vi "NI cDAQ-9188 Producer.vi"(7 "Control Notifier":refnum<notifier>, 8 "error in":errorcluster, 9 "Counter Task":refnum<k21>, 10 "AI Voltage Task":refnum<k21>, 11 "DAQ Notifier":refnum<notifier>) -> (0 "error out":errorcluster, 1 "Counter Task out":refnum<k21>, 2 "AI Voltage Task out":refnum<k21>, 3 "DAQ Notifier out":refnum<notifier>)   [LabVIEW 2013, in "Breakdown Acoustics Controls.lvlib"]
uses:
  Breakdown Acoustics Controls.lvlib
  <vilib>/DAQmx/read.llb/DAQmx Read (Analog 1D Wfm NChan NSamp).vi
  <resource>/objmgr/daqmx.rc
panel:
  in  "Samples per Channel":u32=5120
  in  "Sampling Rate (Hz)":u32=100000
  in  "Stop":bool
  out "ms since last read":u32
  out "Waveform Graph":waveform(dbl)[](graph)
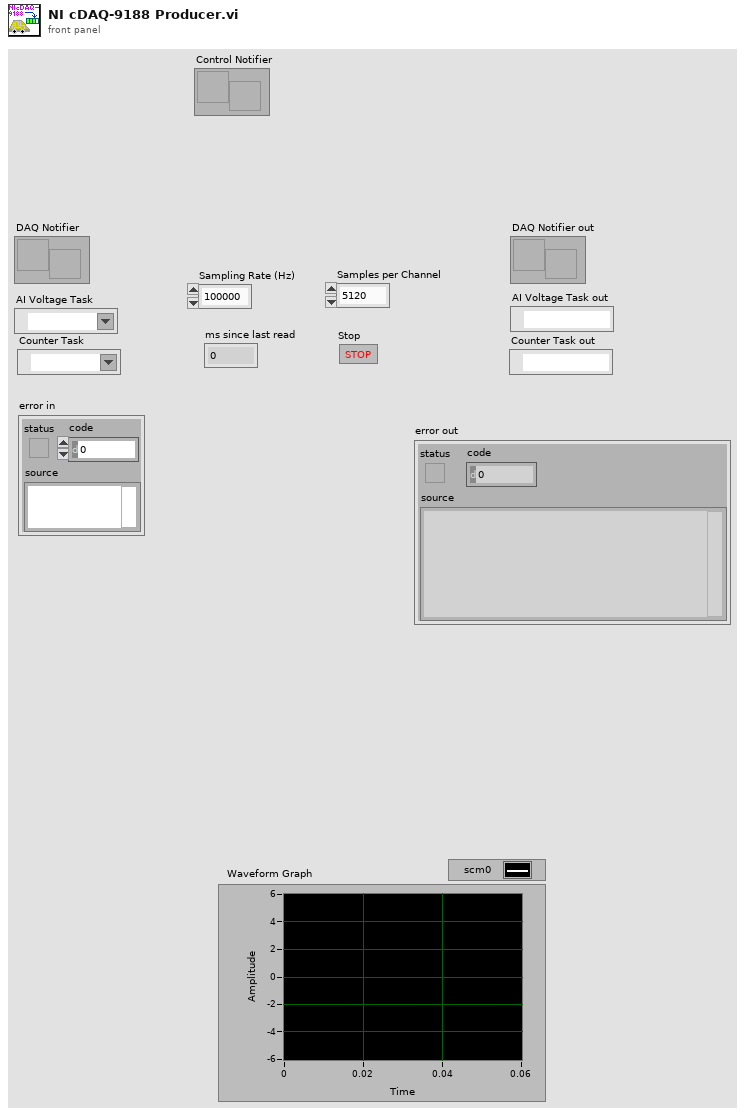
[diagram p1: front panel]
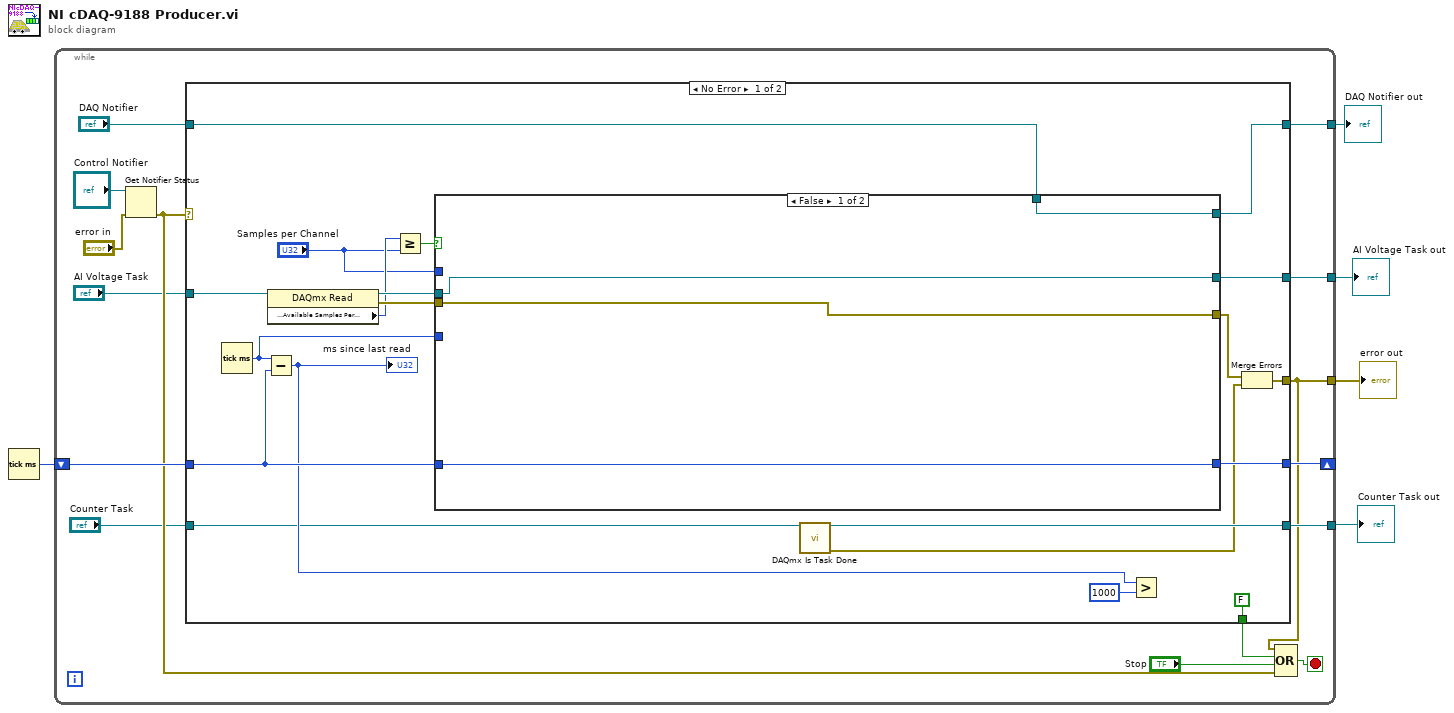
[diagram p0: block diagram]
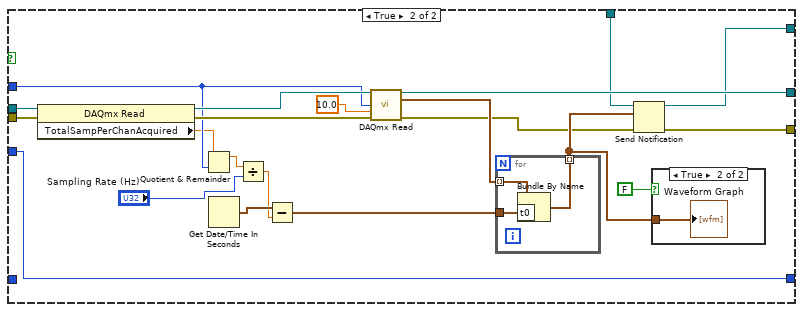
[diagram p2: hidden frame]
diagram:
  n1 = Tick Count (ms)() -> (millisecond timer value=w5:u32)
  n2 = while {
    tunnel: [w20] -> w3
    tunnel: [w19] -> w4
    shift-right: [w17] -> _
    shift-left: w5 -> [w18]
    tunnel: [w12] -> w2
    tunnel: [w6] -> w1
    stop <- w13 stop-if-true
    n3 = Get Notifier Status(notifier="Control Notifier", error in (no error)="error in") -> (error out=w16:errorcluster)  [unwired: 4 out]
    n4 = case shown="No Error" w16 {
      selector: w16 -> [_ w71]
      tunnel: "Counter Task" -> [w24 w72]
      tunnel: [w40 w74] -> w20
      tunnel: [w39 w72] -> w19
      tunnel: "AI Voltage Task" -> [w25 w74]
      tunnel: w18 -> [w34 w73]
      tunnel: [w32 w73] -> w17
      tunnel: [w29 w71] -> w12
      tunnel: [FALSE _] -> w14
      tunnel: [w23 w70] -> w6
      tunnel: "DAQ Notifier" -> [w22 w70]
      frame No Error {
        n5 = Tick Count (ms)() -> (millisecond timer value=w33:u32)
        n6 = Subtract(x=w33, y=w34) -> (x-y=w30:u32)
        "ms since last read" <- w30
        n7 = property class="DAQmx Read"(reference=w25) -> (reference out=w38:refnum<k21>, error out=w37:errorcluster, "Status:Available Samples Per Channel"=w35:u32)  [unwired: 1 in]
        n8 = Greater Or Equal?(x=w35, y="Samples per Channel") -> (x >= y?=w36:bool)
        n9 = case shown="False" w36 {
          tunnel: w38 -> [w43 w65]
          tunnel: w37 -> [w42 w64]
          tunnel: [w43 w57] -> w40
          tunnel: [w42 w47] -> w28
          tunnel: [w44 w63] -> w32
          tunnel: w34 -> [w44 _]
          tunnel: w33 -> [_ w63]
          tunnel: "Samples per Channel" -> [_ w56]
          tunnel: [w41 w46] -> w23
          tunnel: w22 -> [w41 w45]
          frame False {
          }
          frame True {
            n10 = property class="DAQmx Read"(reference=w65, error in=w64) -> (reference out=w61:refnum<k21>, error out=w60:errorcluster, "TotalSampPerChanAcquired"=w54:dbl)
            n11 = Quotient & Remainder(x=w54, y=w56) -> (x-y*floor(x/y)=w53:dbl)  [unwired: 1 out]
            n12 = Get Date/Time In Seconds() -> (seconds since 1Jan1904=w55:timestamp)
            n13 = Divide(x=w53, y="Sampling Rate (Hz)") -> (x/y=w52:dbl)
            n14 = Subtract(x=w55, y=w52) -> (x-y=w59:timestamp)
            n15 = call-poly <vilib>:"DAQmx Read.vi"("task/channels in"=w61, "number of samples per channel"=w56, "timeout"=10.0, "error in"=w60) -> ("task out"=w57:refnum<k21>, "data"=w58:waveform(dbl)[], "error out"=w48:errorcluster)  [unwired: 9 in]
            n16 = for {
              tunnel: w58 -> [w66] mode=indexing
              tunnel: [w68] -> w49 mode=indexing
              tunnel: w59 -> [w67]
              n17 = Bundle By Name(cluster=w66, "t0"=w67) -> (w68:waveform(dbl))
            }
            n18 = Send Notification(notification=w49, notifier=w45, error in (no error)=w48) -> (notifier out=w46:refnum<notifier>, error out=w47:errorcluster)
            n19 = case shown="True" FALSE {
              tunnel: w49 -> [_ w69]
              frame False {
              }
              frame True {
                "Waveform Graph" <- w69
              }
            }
          }
        }
        n20 = call <vilib>:"DAQmx Is Task Done.vi"("task/channels in"=w24) -> ("task out"=w39:refnum<k21>, "error out"=w27:errorcluster)  [unwired: 12 in, 1 out]
        n21 = Greater?(x=w30, y=u32 1000) -> ()  [unwired: 1 out]
        n22 = Merge Errors(w28, w27) -> (w29:errorcluster)
      }
      frame Error {
      }
    }
    n23 = Compound Arithmetic op=OR(w12, w14, "Stop", w16) -> (w13:bool)
  }
  "error out" <- w2
  "Counter Task out" <- w4
  "AI Voltage Task out" <- w3
  "DAQ Notifier out" <- w1
